vi "Parse DB - 1553 - Get RT Config.vi"(0 "channel config handle":u32, 11 "error in (no error)":errorcluster) -> (4 "channel config handle out":u32, 8 "RT_Messages":T1[](array[typedef]), 15 "error out":errorcluster)   [LabVIEW 2013, in "AIT 1553 Custom Device.lvlib"]
uses:
  AIT 1553 Custom Device.lvlib
  Controls/1553_RT_Message.ctl
  Controls/1553 Param.ctl
  <userlib>/MIL-STD-1553/Owl1553.lvlib
panel:
  out "RT Tx Array":bool[][](array[boolean])
  out "RT Rx Array":bool[][](array[boolean])
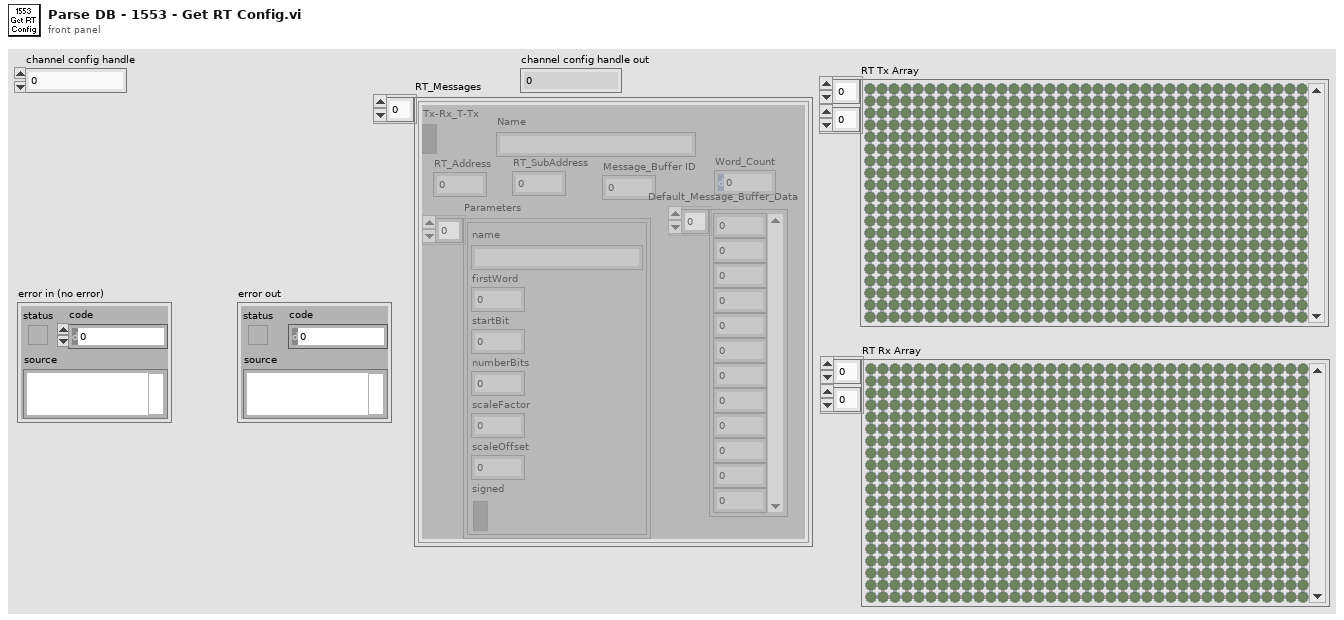
[diagram p1: front panel]
types:
  T1 = typedef "AIT 1553 Custom Device.lvlib/1553_RT_Message.ctl" = cluster{"RT_Address":u8, "RT_SubAddress":u8, "Tx-Rx_T-Tx":bool, "Parameters":T2[], "Message_Buffer ID":u16, "Default_Message_Buffer_Data":u16[], "Word_Count":u8, "Name":string}
  T2 = typedef "AIT 1553 Custom Device.lvlib/1553 Param.ctl" = cluster{"name":string, "firstWord":i32, "startBit":i32, "numberBits":i32, "scaleFactor":dbl, "scaleOffset":dbl, "signed":bool}
  T3 = enum16{"OWL1553_RECEIVE_TRANSFER", "OWL1553_TRANSMIT_TRANSFER"}
  T4 = enum16{"OWL_1553_MILBUS_CHANNEL_PRIMARY", "OWL_1553_MILBUS_CHANNEL_SECONDARY"}
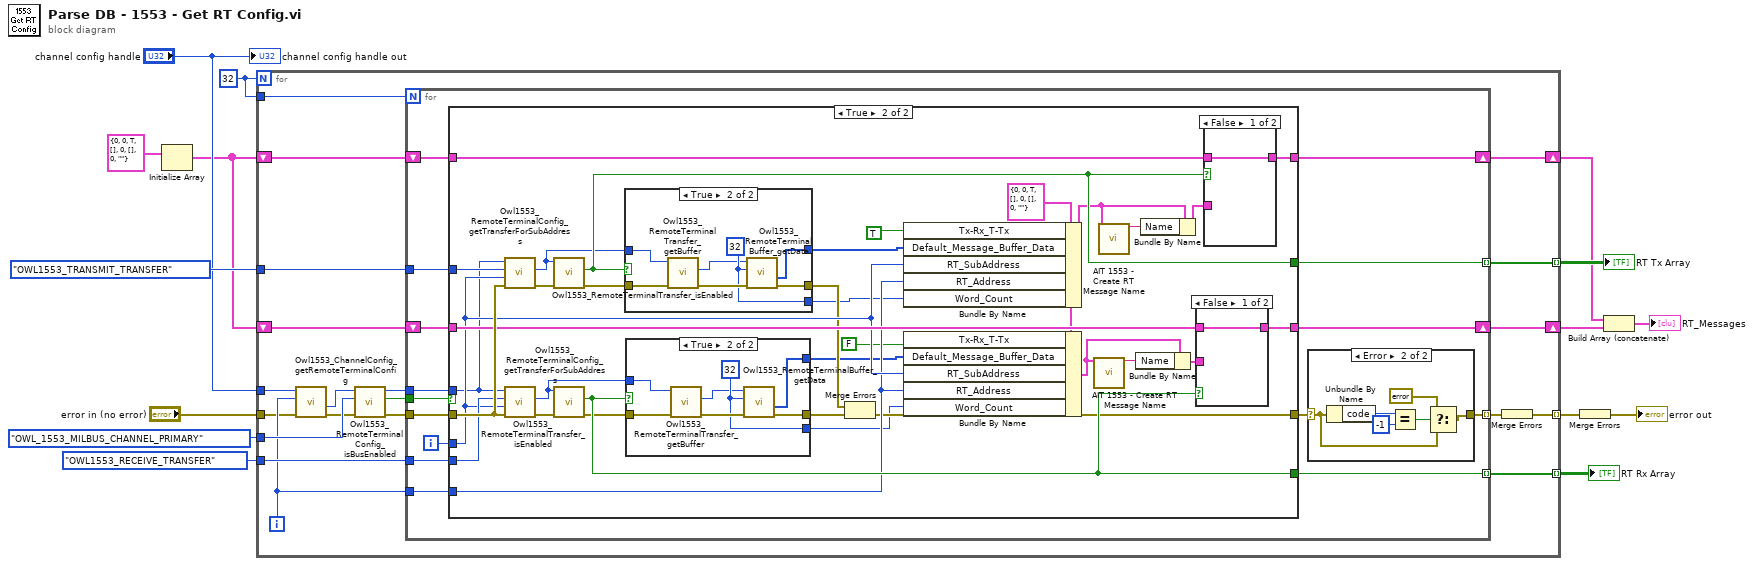
[diagram p0: block diagram]
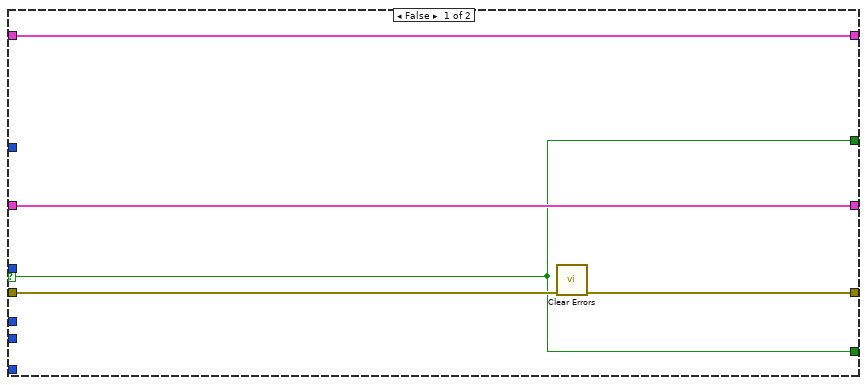
[diagram p3: hidden frame]
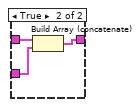
[diagram p4: hidden frame]
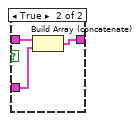
[diagram p6: hidden frame]
diagram:
  w11 = 32
  n1 = Initialize Array(T1 {"RT_Address"=0, "RT_SubAddress"=0, "Tx-Rx_T-Tx"=TRUE, "Parameters"=[], "Message_Buffer ID"=0, "Default_Message_Buffer_Data"=[], "Word_Count"=0, "Name"=""} ("RT_Message")) -> (w4:T1[])  [unwired: 1 in]
  n2 = for {
    N: w11 -> [_]
    tunnel: T4."OWL_1553_MILBUS_CHANNEL_PRIMARY" ("milbus") -> [w34]
    tunnel: "channel config handle" -> [w35]
    tunnel: w11 -> [w30]
    tunnel: [w29] -> w9 mode=indexing
    tunnel: T3."OWL1553_TRANSMIT_TRANSFER" ("direction") -> [w27]
    tunnel: T3."OWL1553_RECEIVE_TRANSFER" ("direction") -> [w26]
    tunnel: [w25] -> w10 mode=indexing
    shift-right: [w24] -> w7
    shift-left: w4 -> [w23]
    shift-right: [w21] -> w8
    shift-left: w4 -> [w22]
    tunnel: "error in (no error)" -> [w17]
    tunnel: [w16] -> w2 mode=indexing
    i -> [w20]
    n3 = call <userlib>:"Owl1553_ChannelConfig_getRemoteTerminalConfig.vi"("error in (no error)"=w17, "remote terminal"=w20, "channel config handle"=w35) -> ("error out"=w33:errorcluster, "remote terminal config handle"=w32:u32)  [unwired: 5 in, 2 out]
    n4 = call <userlib>:"Owl1553_RemoteTerminalConfig_isBusEnabled.vi"("error in (no error)"=w33, "milbus"=w34, "remote terminal config handle"=w32) -> ("error out"=w19:errorcluster, "is enabled"=w31:bool, "remote terminal config handle"=w28:u32)  [unwired: 6 in]
    n5 = for {
      N: w30 -> [_]
      tunnel: w31 -> [w50]
      tunnel: [w49] -> w29 mode=indexing
      tunnel: w28 -> [w48]
      tunnel: w27 -> [w47]
      tunnel: w26 -> [w46]
      tunnel: [w45] -> w25 mode=indexing
      shift-right: [w44] -> w24
      shift-left: w23 -> [w43]
      shift-right: [w41] -> w21
      shift-left: w22 -> [w42]
      tunnel: w20 -> [w39]
      tunnel: w19 -> [w38]
      tunnel: [w36] -> w18 mode=indexing
      i -> [w40]
      n6 = case shown="True" w50 {
        selector: w50 -> [w58 _]
        tunnel: [w61 w78] -> w37
        tunnel: w38 -> [w62 w93]
        tunnel: [w58 w87] -> w49
        tunnel: w48 -> [_ w82]
        tunnel: w40 -> [_ w83]
        tunnel: w47 -> [_ w96]
        tunnel: w46 -> [_ w84]
        tunnel: [w58 w86] -> w45
        tunnel: [w60 w91] -> w44
        tunnel: w43 -> [w60 w92]
        tunnel: w42 -> [w59 w90]
        tunnel: [w59 w89] -> w41
        tunnel: w39 -> [_ w81]
        frame False {
          n7 = call <vilib>:"Clear Errors.vi"("error in (no error)"=w62) -> ("error out"=w61:errorcluster)  [unwired: 6 in]
        }
        frame True {
          w75 = T1 {"RT_Address"=0, "RT_SubAddress"=0, "Tx-Rx_T-Tx"=TRUE, "Parameters"=[], "Message_Buffer ID"=0, "Default_Message_Buffer_Data"=[], "Word_Count"=0, "Name"=""} ("RT_Message")
          n8 = call <userlib>:"Owl1553_RemoteTerminalConfig_getTransferForSubAddress.vi"("error in (no error)"=w93, "sub address"=w83, "direction"=w96, "remote terminal config handle"=w82) -> ("error out"=w95:errorcluster, "transfer handle"=w69:u32)  [unwired: 5 in, 1 out]
          n9 = call <userlib>:"Owl1553_RemoteTerminalConfig_getTransferForSubAddress.vi"("error in (no error)"=w93, "sub address"=w83, "direction"=w84, "remote terminal config handle"=w82) -> ("error out"=w94:errorcluster, "transfer handle"=w70:u32)  [unwired: 5 in, 1 out]
          n10 = call <userlib>:"Owl1553_RemoteTerminalTransfer_isEnabled.vi"("error in (no error)"=w95, "remote terminal transfer handle"=w69) -> ("error out"=w88:errorcluster, "is enabled"=w87:bool)  [unwired: 7 in, 1 out]
          n11 = call <userlib>:"Owl1553_RemoteTerminalTransfer_isEnabled.vi"("error in (no error)"=w94, "remote terminal transfer handle"=w70) -> ("error out"=w85:errorcluster, "is enabled"=w86:bool)  [unwired: 7 in, 1 out]
          n12 = case shown="True" w87 {
            tunnel: w88 -> [w113 w118]
            tunnel: [w113 w120] -> w80
            tunnel: [_ w119] -> w76
            tunnel: [_ w115] -> w72
            tunnel: w69 -> [_ w117]
            frame False {
            }
            frame True {
              w115 = u32 32
              n13 = call <userlib>:"Owl1553_RemoteTerminalTransfer_getBuffer.vi"("error in (no error)"=w118, "remote terminal transfer handle"=w117) -> ("error out"=w116:errorcluster, "buffer"=w114:u32)  [unwired: 7 in, 1 out]
              n14 = call <userlib>:"Owl1553_RemoteTerminalBuffer_getData.vi"("error in (no error)"=w116, "buffer size"=w115, "buffer handle"=w114) -> ("error out"=w120:errorcluster, "data"=w119:u16[])  [unwired: 5 in, 2 out]
            }
          }
          n15 = case shown="True" w86 {
            tunnel: w85 -> [w101 w106]
            tunnel: [w101 w108] -> w79
            tunnel: [_ w102] -> w77
            tunnel: [_ w104] -> w71
            tunnel: w70 -> [_ w107]
            frame False {
            }
            frame True {
              w104 = u32 32
              n16 = call <userlib>:"Owl1553_RemoteTerminalTransfer_getBuffer.vi"("error in (no error)"=w106, "remote terminal transfer handle"=w107) -> ("error out"=w105:errorcluster, "buffer"=w103:u32)  [unwired: 7 in, 1 out]
              n17 = call <userlib>:"Owl1553_RemoteTerminalBuffer_getData.vi"("error in (no error)"=w105, "buffer size"=w104, "buffer handle"=w103) -> ("error out"=w108:errorcluster, "data"=w102:u16[])  [unwired: 5 in, 2 out]
            }
          }
          n18 = Merge Errors(w80, w79) -> (w78:errorcluster)
          n19 = Bundle By Name(cluster=w75, "Tx-Rx_T-Tx"=TRUE ("Tx-Rx (T=Tx)"), "Default_Message_Buffer_Data"=w76, "RT_SubAddress"=w83, "RT_Address"=w81, "Word_Count"=w72) -> (w68:T1)
          n20 = Bundle By Name(cluster=w75, "Tx-Rx_T-Tx"=FALSE ("Tx-Rx (T=Tx)"), "Default_Message_Buffer_Data"=w77, "RT_SubAddress"=w83, "RT_Address"=w81, "Word_Count"=w71) -> (w64:T1)
          n21 = call "AIT 1553 - Create RT Message Name.vi"("RT_Message"=w64) -> ("Message Name"=w65:string)  [unwired: 13 in, 1 out]
          n22 = call "AIT 1553 - Create RT Message Name.vi"("RT_Message"=w68) -> ("Message Name"=w66:string)  [unwired: 13 in, 1 out]
          n23 = Bundle By Name(cluster=w64, "Name"=w65) -> (w63:T1)
          n24 = Bundle By Name(cluster=w68, "Name"=w66) -> (w67:T1)
          n25 = case shown="False" w86 {
            tunnel: w90 -> [w97 w100]
            tunnel: w63 -> [_ w99]
            tunnel: [w97 w98] -> w89
            frame False {
            }
            frame True {
              n26 = Build Array (concatenate)(w100, w99) -> (w98:T1[])
            }
          }
          n27 = case shown="False" w87 {
            tunnel: w92 -> [w109 w112]
            tunnel: w67 -> [_ w111]
            tunnel: [w109 w110] -> w91
            frame False {
            }
            frame True {
              n28 = Build Array (concatenate)(w112, w111) -> (w110:T1[])
            }
          }
        }
      }
      n29 = case shown="Error" w37 {
        selector: w37 -> [w51 w55]
        tunnel: [w51 w52] -> w36
        frame No Error {
        }
        frame Error {
          n30 = Unbundle By Name(w55) -> ("code"=w57:i32)
          n31 = Equal?(x=w57, y=-1) -> (x = y?=w54:bool)
          n32 = Select(t=errorcluster {"status"=FALSE, "code"=0, "source"=""}, s=w54, f=w55) -> (s? t:f=w52:errorcluster)
        }
      }
    }
    n33 = Merge Errors(w18) -> (w16:errorcluster)
  }
  "RT Tx Array" <- w9
  "RT Rx Array" <- w10
  n34 = Merge Errors(w2) -> (→"error out":errorcluster)
  n35 = Build Array (concatenate)(w7, w8) -> (→"RT_Messages":T1[])
  "channel config handle out" <- "channel config handle"
